vi "Measurement.IVCurve.UI.GetDependencies.vi"(8 "error in (no error)":errorcluster, 11 "Measurement.IVCurve.UI in":refnum<class "Measurement.IVCurve.UI.lvclass">) -> (0 "error out":errorcluster, 2 "Dependencies":T1, 3 "Measurement.IVCurve.UI out":refnum<class "Measurement.IVCurve.UI.lvclass">)   [LabVIEW 2017, in "Measurement.IVCurve.UI.lvclass"]
uses:
  Measurement.IVCurve.UI.lvclass
  Typedefs/Dependencies--Cluster.ctl
  Measurement.IVCurve/Measurement.IVCurve.lvclass
  Measurement.IVCurve.UI.lvclass/Measurement.IVCurve.UI.ctl
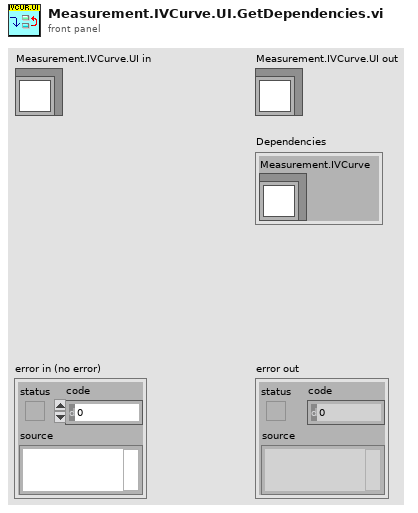
[diagram p1: front panel]
types:
  T1 = typedef "Measurement.IVCurve.UI.lvclass/Dependencies--Cluster.ctl" = cluster{"Measurement.IVCurve":refnum<class "Measurement.IVCurve.lvclass">}
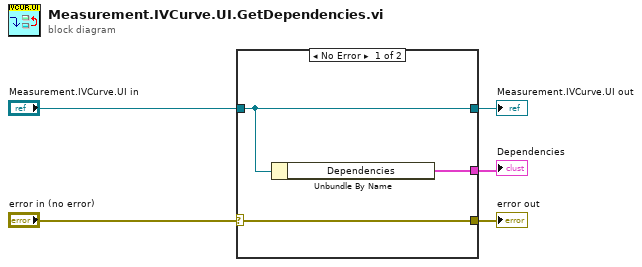
[diagram p0: block diagram]
diagram:
  n1 = case shown="No Error" "error in (no error)" {
    selector: "error in (no error)" -> [w8 w10]
    tunnel: [w8 w10] -> w4
    tunnel: [w7 w9] -> w2
    tunnel: "Measurement.IVCurve.UI in" -> [w7 w9]
    tunnel: [w6 _] -> w1
    frame No Error {
      n2 = Unbundle By Name(w7) -> ("Dependencies"=w6:T1)
    }
    frame Error {
    }
  }
  "error out" <- w4
  "Measurement.IVCurve.UI out" <- w2
  "Dependencies" <- w1
